vi "Array&Matrix&Waveform.vi"() -> ()   [LabVIEW 2024]
uses:
  <vilib>/Analysis/baseanly.llb/Real A x B.vi
  <vilib>/Analysis/NI_AALBase.lvlib
panel:
  in  "Origin":dbl[](array[numeric])
  out "F 3":dbl[](array[numeric])
  in  "C3":dbl[](array[numeric])
  out "Transferd Array F = A x C":dbl[][](array[numeric])
  in  "Transfer Matrix A":dbl[][](array[numeric])
  out "Force Data":waveform(dbl)[](graph)
  out "F2":dbl[](array[numeric])
  out "F1":dbl[](array[numeric])
  out "Input Array C-Origin":dbl[][](array[numeric])
  in  "C 2":dbl[](array[numeric])
  in  "C1":dbl[](array[numeric])
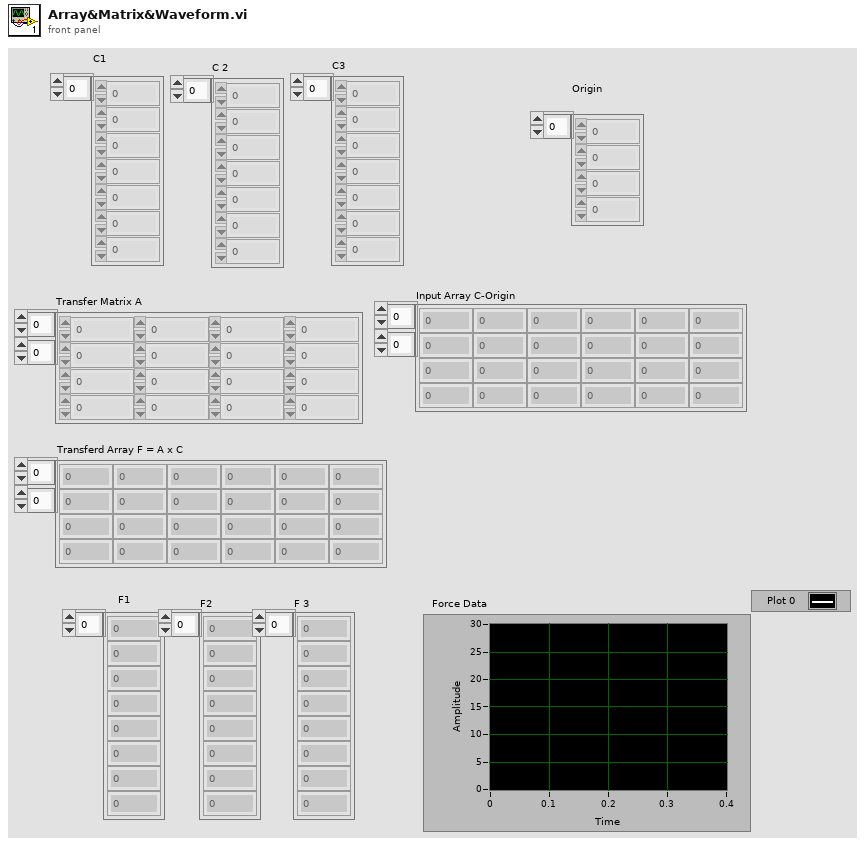
[diagram p1: front panel]
types:
  T1 = typedef "NI_Matrix.lvlib/RealMatrix.ctl" = dbl[][]
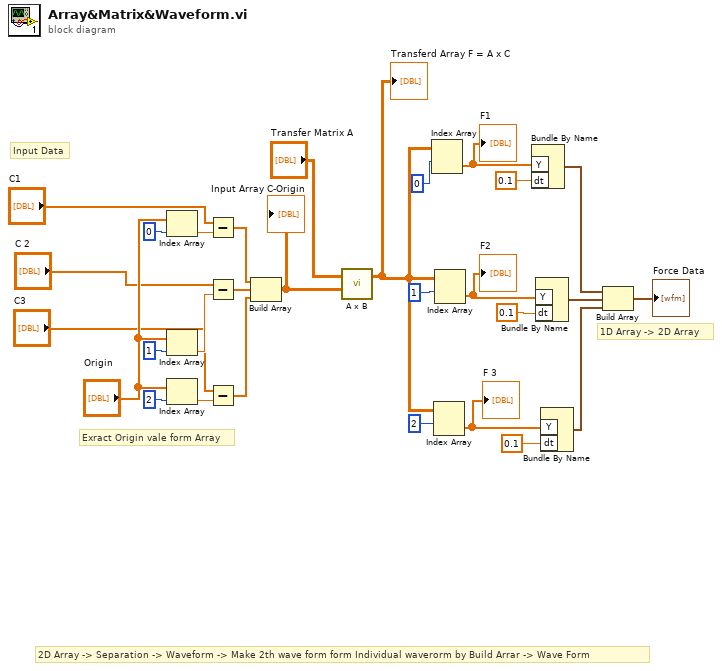
[diagram p0: block diagram]
diagram:
  # "Exract Origin vale form Array"
  # "Input Data"
  # "2D Array -> Separation -> Waveform -> Make 2th wave form form Individual waverorm by Build Arrar -> Wave Form"
  # "1D Array -> 2D Array"
  n1 = Index Array(array="Origin", index=0) -> (element=w8:dbl)
  n2 = Index Array(array="Origin", index=1) -> (element=w7:dbl)
  n3 = Index Array(array="Origin", index=2) -> (element=w6:dbl)
  n4 = Subtract(x="C1", y=w8) -> (x-y=w13:dbl[])
  n5 = Subtract(x="C 2", y=w7) -> (x-y=w2:dbl[])
  n6 = Subtract(x="C3", y=w6) -> (x-y=w3:dbl[])
  n7 = Build Array(w13, w2, w3) -> (w15:dbl[][])
  "Input Array C-Origin" <- w15
  n8 = call-poly <vilib>:"A x B.vi"("B"=w15, "A"="Transfer Matrix A") -> ("A x B"=w1:T1)  [unwired: 1 out]
  "Transferd Array F = A x C" <- w1
  n9 = Index Array(array=w1, index (row)=0) -> (element=w27:dbl[])  [unwired: 1 in]
  "F1" <- w27
  n10 = Index Array(array=w1, index (row)=2) -> (element=w17:dbl[])  [unwired: 1 in]
  "F 3" <- w17
  n11 = Index Array(array=w1, index (row)=1) -> (element=w24:dbl[])  [unwired: 1 in]
  "F2" <- w24
  n12 = Bundle By Name("Y"=w27, "dt"=0.1) -> (w23:waveform(dbl))  [unwired: 1 in]
  n13 = Bundle By Name("Y"=w24, "dt"=0.1) -> (w22:waveform(dbl))  [unwired: 1 in]
  n14 = Bundle By Name("Y"=w17, "dt"=0.1) -> (w16:waveform(dbl))  [unwired: 1 in]
  n15 = Build Array(w23, w22, w16) -> (→"Force Data":waveform(dbl)[])
